vi "crio_RT_VCA.vi"() -> ()   [LabVIEW 2019]
uses:
  <vilib>/Platform/TimedLoop/XDataNode/timing_clust.ctl
  <vilib>/Platform/TimedLoop/XDataNode/nitl_modes.ctl
  <vilib>/Platform/TimedLoop/XDataNode/wakeup.ctl
  <vilib>/FPGAPlugInAG/cRIO-9074/niLvFpga_Open_cRIO-9074.vi
  <vilib>/rvi/interface/common/dynamic/niFpgaDynamicAddResources.vi
  <vilib>/Utility/error.llb/Error Cluster From Error Code.vi
  <vilib>/rvi/errors/niLvFpgaAdjustHostInterfaceError.vi
  <vilib>/FPGAPlugInAG/Dynamic/niLvFpga_Close_Dynamic.vi
  <vilib>/rvi/interface/nirviOpenFPGA/nirviOpenFPGA.xnode
  FPGA Bitfiles/gpass2_FPGATarget2_crioFPGAPWMeffic_pZbzPKfzVSQ.lvbitx
  crio_FPGA_PWM_efficient.vi
  <vilib>/rvi/interface/nirviReadWriteControl/nirviReadWriteControl.xnode
  <vilib>/platform/TimedLoop/XDataNode/XDataNode.xnode
  <vilib>/rvi/interface/nirviCloseFPGA/nirviCloseFPGA.xnode
  NiFpgaLv.dll
  <vilib>/rvi/interface/Simulation/niFpgaSimulationCallBeginRW.vi
  <vilib>/Platform/TimedLoop/XDataNode/XDNodeRunTimeDep.lvlib
panel:
  in  "Offset":dbl
  in  "Frequency":dbl=10.1
  in  "Amplitude":dbl=1.0
  out "setpoint":i32(slide)=2000 scale=0.0..2700.0
  in  "Enum":enum16{"sine", "manual"}(ring)
  in  "Gain Scaler":T1={"proportional gain"=1000.0, "integral gain"=100000000.0}
  out "Actual Gain":T1={"proportional gain"=0.0009797979, "integral gain"=5.30303e-09}
  in  "manual setpoint":i32(slide)=2000 scale=0.0..2700.0
  out "measured position":i64(graph)=2000
  out "Measured Position":i64=2000
  out "Controller PWM Output":sgl=0.1282059
  out "Measured Velocity (Counts/Interval)":i32
  out "velocity":i32(graph)
  out "controller pwm output":sgl(graph)=0.1282059
  in  "Velocity Interval (uSec)":u32=1000
  in  "Gains":T1={"proportional gain"=0.97979796, "integral gain"=0.530303} {"proportional gain" scale=0.0..1.0; "integral gain" scale=0.0..1.0}
  in  "Position Reset":bool
  in  "manual control":T2 {"manual input (0)" scale=-1.0..1.0}
  in  "stop":bool=TRUE
  in  "Loop Period":i64=1000
  in  "PWM Frequency (default 20kHz)":i32=20000
  # "2700 is about fully stretched"
  # "100us = 10kHz"
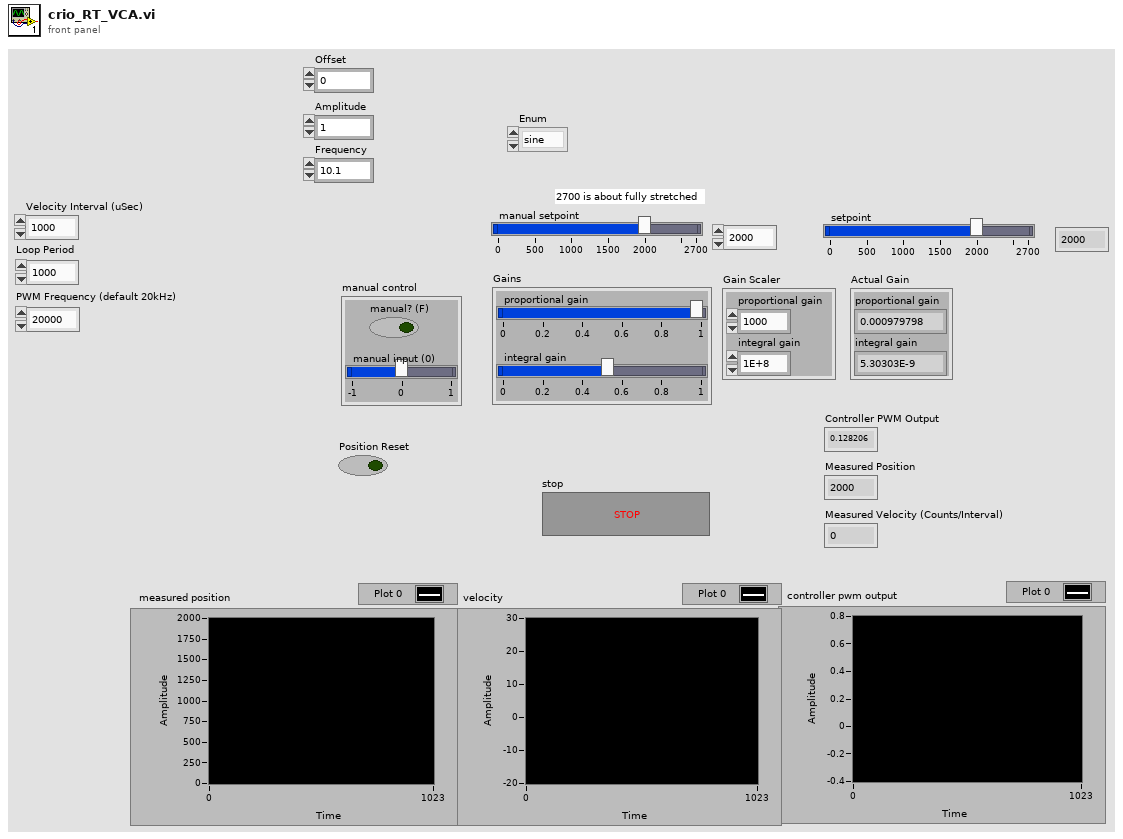
[diagram p1: front panel]
types:
  T1 = cluster{"proportional gain":sgl, "integral gain":sgl}
  T2 = cluster{"manual? (F)":bool, "manual input (0)":sgl}
  T3 = typedef "XDNodeRunTimeDep.lvlib/timing_clust.ctl" = cluster{"Expected End [f-1]":u64, "Actual End [f-1]":u64, "Finished Late? [f-1]":bool, "Expected End [i-1]":u64, "Actual End [i-1]":u64, "Finished Late? [i-1]":bool, "Expected Start [i]":u64, "Actual Start [i]":u64, "Expected Start [f]":u64, "Actual Start [f]":u64, "Source Name":string, "Structure Name":string, "Period":i64, "Deadline":i64, "Offset":i64, "Start":i64, "Priority":i32, "Timeout":i32, "Mode":T4, "Wakeup Reason":T5, "Error":errorcluster, "Source Type":string, "Secondary Source Type":string, "Global End Time":u64, "Global Start Time":u64, "Frame Duration":u64, "Iteration Duration":u64, "Assigned CPU":i32, "I/O Scan Engine Mode":u32}
  T4 = typedef "XDNodeRunTimeDep.lvlib/nitl_modes.ctl" = enum32{"No Change", "Process missed periods, maintain original phase", "Discard missed periods, maintain original phase", "Process missed periods, ignore original phase", "Discard missed periods, ignore original phase"}
  T5 = typedef "XDNodeRunTimeDep.lvlib/wakeup.ctl" = enum32{"Normal", "Aborted", "Asynchronous wakeup", "Timing source error", "Timed loop error", "Timeout"}
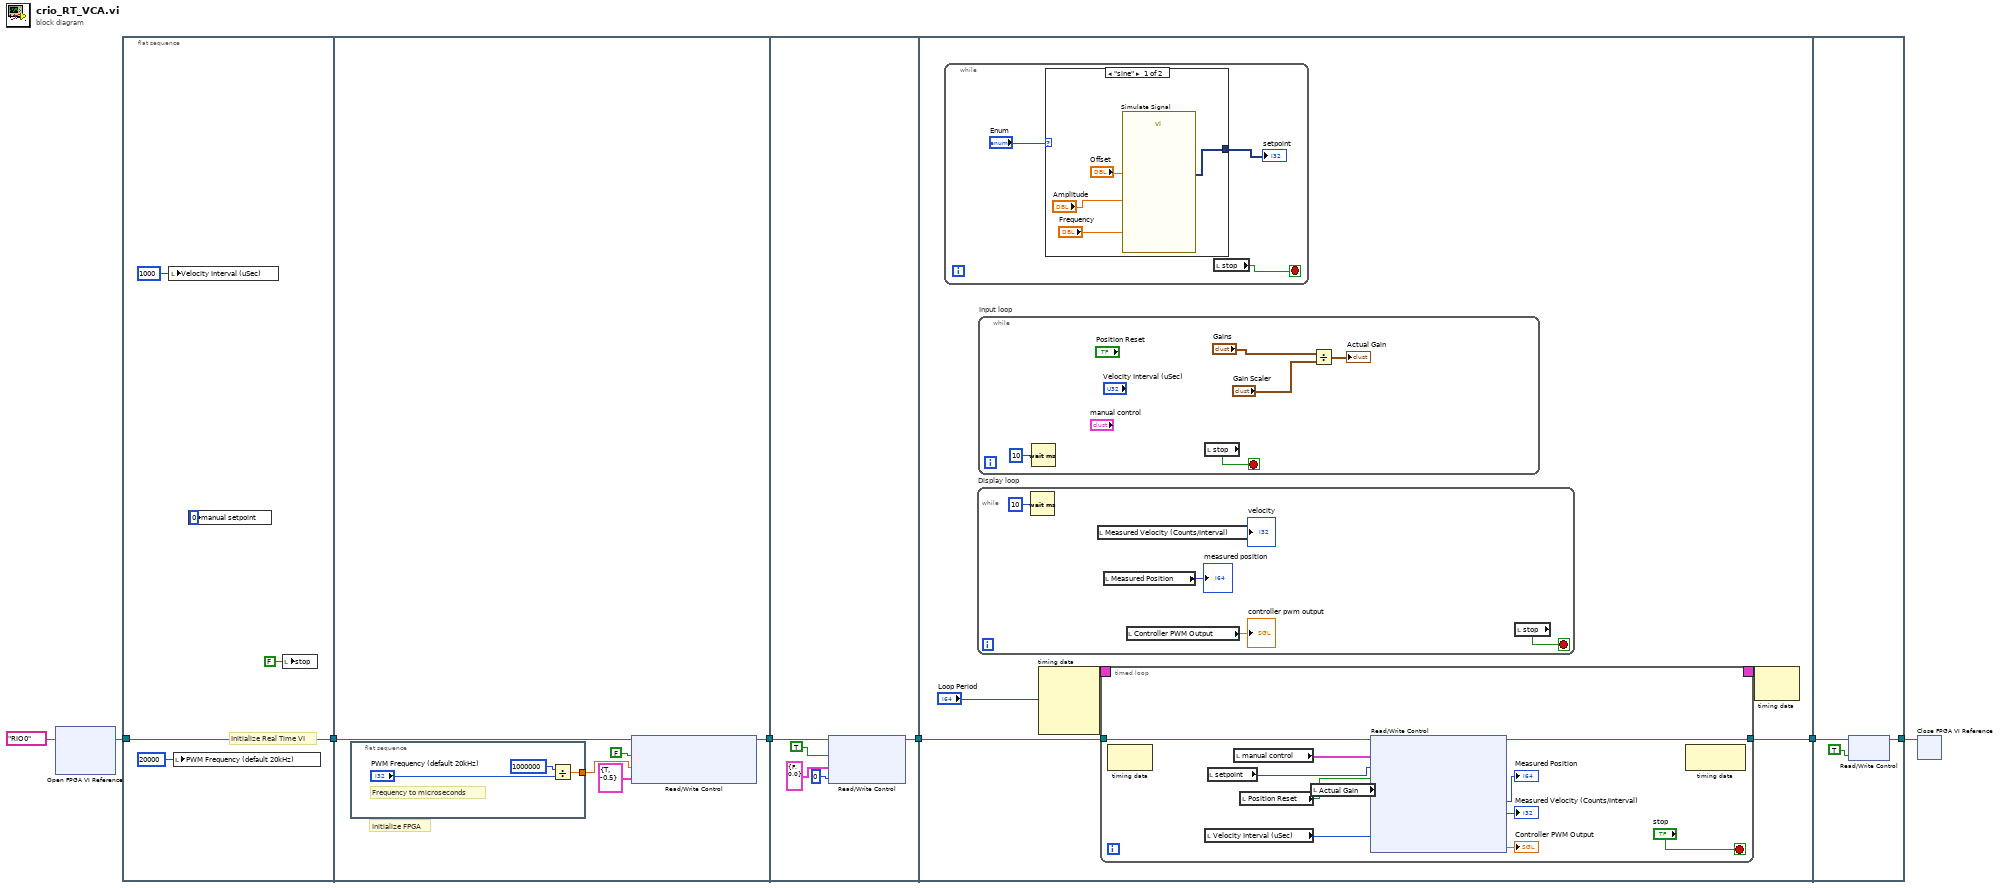
[diagram p0: block diagram]
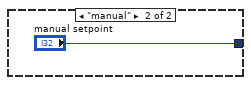
[diagram p2: hidden frame]
diagram:
  n1 = xnode "Open FPGA VI Reference"("resource name"=tag "RIO0") -> ("FPGA VI Reference Out"=w5:refnum<k20>)  [unwired: 1 in, 1 out]
  n2 = flat-sequence {
    tunnel: [w11] -> w6
    tunnel: w5 -> [w11]
    tunnel: w6 -> [w16]
    tunnel: [w14] -> w4
    tunnel: w4 -> [w24]
    tunnel: [w25] -> w3
    tunnel: w3 -> [w27]
    tunnel: [w26] -> w2
    tunnel: w2 -> [w68]
    tunnel: [w66] -> w1
    frame #0 {
      # "Initialize Real Time VI"
      n3 = local write "Velocity Interval (uSec)"(u32 1000 ("Velocity Interval (uSec)")) -> ()
      n4 = local write "PWM Frequency (default 20kHz)"(20000 ("PWM Frequency")) -> ()
      n5 = local write "manual setpoint"(0 ("setpoint")) -> ()
      n6 = local write "stop"(FALSE ("stop")) -> ()
    }
    frame #1 {
      # "Initialize FPGA"
      n7 = flat-sequence {
        tunnel: [w18] -> w15
        frame #0 {
          # "Frequency to microseconds"
          n8 = Divide(x=1000000, y="PWM Frequency (default 20kHz)") -> (x/y=w18:dbl)
        }
      }
      n9 = xnode "Read/Write Control"("FPGA VI Reference In"=w16, "stop"=FALSE, "DC PWM Period (microsec)"=w15, "manual control"=T2 {"manual? (F)"=TRUE, "manual input (0)"=-0.5}) -> ("FPGA VI Reference Out"=w14:refnum<k20>)  [unwired: 1 in, 1 out]
    }
    frame #2 {
      n10 = xnode "Read/Write Control"("FPGA VI Reference In"=w24, "Position Reset"=TRUE, "manual control"=T2 {"manual? (F)"=FALSE, "manual input (0)"=0.0}, "setpoint"=0) -> ("FPGA VI Reference Out"=w25:refnum<k20>)  [unwired: 1 in, 1 out]
    }
    frame #3 {
      n11 = while {
        stop <- w31 stop-if-true
        n12 = case shown="\"sine\"" "Enum" {
          tunnel: [w36 "manual setpoint"] -> w32
          frame "sine" {
            n13 = call "Simulate Signal"("Offset"="Offset", "Frequency"="Frequency", "Amplitude"="Amplitude") -> ("Sine"=w36:dynamicdata)  [unwired: 11 in, 1 out]
          }
          frame "manual" {
          }
        }
        "setpoint" <- w32
        n14 = local read "stop"() -> (w31:bool)
      }
      n15 = while "Display loop" {
        stop <- w47 stop-if-true
        n16 = Wait (ms)(milliseconds to wait=u32 10) -> ()  [unwired: 1 out]
        n17 = local read "Measured Velocity (Counts/Interval)"() -> (→"velocity":i32)
        n18 = local read "Measured Position"() -> (→"measured position":i64)
        n19 = local read "Controller PWM Output"() -> (→"controller pwm output":sgl)
        n20 = local read "stop"() -> (w47:bool)
      }
      n21 = while "Input loop" {
        stop <- w42 stop-if-true
        n22 = Wait (ms)(milliseconds to wait=u32 10) -> ()  [unwired: 1 out]
        n23 = local read "stop"() -> (w42:bool)
        n24 = Divide(x="Gains", y="Gain Scaler") -> (x/y=→"Actual Gain":T1)
      }
      n25 = node-c288("Loop Period") -> (w30:T3)  [unwired: 3 in]
      n26 = timed-loop {
        timing: w30 -> [_]
        timing-out: [_] -> w29
        tunnel: w27 -> [w58]
        tunnel: [w50] -> w26
        stop <- "stop" stop-if-true
        n27 = node-c288() -> ()  [unwired: 1 in, 1 out]
        n28 = local read "Velocity Interval (uSec)"() -> (w51:u32)
        n29 = local read "setpoint"() -> (w49:i32)
        n30 = local read "manual control"() -> (w52:T2)
        n31 = local read "Position Reset"() -> (w54:bool)
        n32 = local read "Actual Gain"() -> (w53:T1)
        n33 = xnode "Read/Write Control"("FPGA VI Reference In"=w58, "manual control"=w52, "setpoint"=w49, "Position Reset"=w54, "gains"=w53, "Velocity Interval (uSec)"=w51) -> ("FPGA VI Reference Out"=w50:refnum<k20>, "Position (Counts)"=→"Measured Position":i32, "Velocity (Counts/Interval)"=→"Measured Velocity (Counts/Interval)":i32, "ControllerPWM Output"=→"Controller PWM Output":sgl)  [unwired: 1 in, 2 out]
        n34 = node-c288() -> ()  [unwired: 1 in, 1 out]
      }
      n35 = node-c288(w29) -> ()  [unwired: 1 out]
    }
    frame #4 {
      n36 = xnode "Read/Write Control"("FPGA VI Reference In"=w68, "stop"=TRUE) -> ("FPGA VI Reference Out"=w66:refnum<k20>)  [unwired: 1 in, 1 out]
    }
  }
  n37 = xnode "Close FPGA VI Reference"("FPGA VI Reference In"=w1) -> ()  [unwired: 1 in, 1 out]
